vi "GryoEngine.vi"(11 "Gyro_Zero":bool) -> (3 "GyroData":T1)   [LabVIEW 2017]
uses:
  Support Code/Gyro/Gyro_TypeDef.ctl
  Framework/Robot Global Data.vi
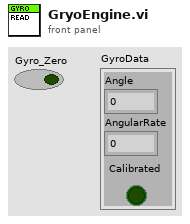
[diagram p1: front panel]
types:
  T1 = typedef "Gyro_TypeDef.ctl" = cluster{"Angle":dbl, "AngularRate":dbl, "Calibrated":bool}
  T2 = typedef "WPI_GyroDevRef.ctl" = cluster{"DevStatus":errorcluster, "Analog Channel":T3, "Gain (VoltsPerDegree/Second)":dbl, "Gyro Type":enum16{"Analog", "XRS450"}, "Handle":i32, "SPI Bus":T4, "Device Found":bool, "Sample Rate":dbl, "Calibrate On Open":bool, "Offset":dbl}
  T3 = typedef "FPGA_AIChannel.ctl" = enum8{"AI 0", "AI 1", "AI 2", "AI 3", "AI MXP 0", "AI MXP 1", "AI MXP 2", "AI MXP 3", "Invalid"}
  T4 = typedef "spi_bus.ctl" = enum16{"SPI On-Board, CS0", "SPI On-Board, CS1", "SPI On-Board, CS2", "SPI On-Board, CS3", "SPI MXP", "Invalid"}
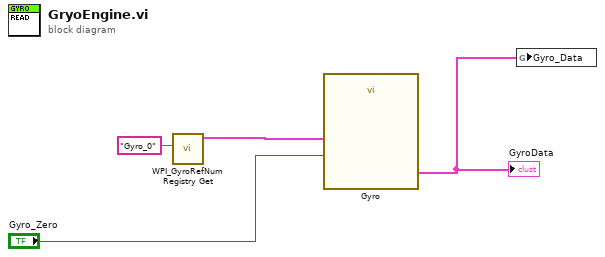
[diagram p0: block diagram]
diagram:
  n1 = call <vilib>:"WPI_GyroRefNum Registry Get.vi"("refnum name"="Gyro_0") -> ("GyroDevRef"=w3:T2)  [unwired: 9 in, 1 out]
  n2 = call "Gyro.vi"("ResetAngle"="Gyro_Zero", "GyroDevRef"=w3) -> ("GyroData"=w1:T1)  [unwired: 7 in]
  "GyroData" <- w1
  n3 = global write "Robot Global Data.vi" "Gyro_Data"(w1) -> ()
